vi "OpenProject1.vi"() -> ()   [LabVIEW 2020]
uses:
  <vilib>/Wiresmith Technology/G CLI/CLI Class/CLI.lvclass
  <vilib>/addons/_JKI Toolkits/Caraya/classes/Test Runner/Test Runner.lvclass/Test Runner.ctl
  <vilib>/Wiresmith Technology/G CLI/CLI Class/Output.ctl
  <vilib>/addons/_JKI Toolkits/Caraya/classes/Test Report.JUnit/Test Report.JUnit.lvclass
  C:/Program Files/National Instruments/LabVIEW 2020/vi.lib/addons/_JKI Toolkits/Caraya/classes/Test Report/Test Report.lvclass
  <vilib>/addons/_JKI Toolkits/Caraya/classes/Test Runner.Project/Test Runner.Project.lvclass
  C:/Program Files/National Instruments/LabVIEW 2020/vi.lib/addons/_JKI Toolkits/Caraya/classes/Test Runner/Test Runner.lvclass
  <vilib>/addons/_JKI Toolkits/Caraya/classes/Test Suite/Define Test Suite (Default).vi
  <vilib>/addons/_JKI Toolkits/Caraya/classes/Test Suite/Test Suite.lvclass
  <vilib>/addons/_JKI Toolkits/Caraya/classes/Test Runner/Test Runner.lvclass
  C:/Program Files/National Instruments/LabVIEW 2020/vi.lib/addons/_JKI Toolkits/Caraya/classes/Test Report.JUnit/Test Report.JUnit.lvclass
panel:
  in  "Report Path":path
  in  "Error in":errorcluster
  in  "CLI":refnum<class "CLI.lvclass">
  in  "Project Reference":refnum<vi>
  in  "Virtual Folder (empty: \"My Computer\")":string
  out "Error out":errorcluster
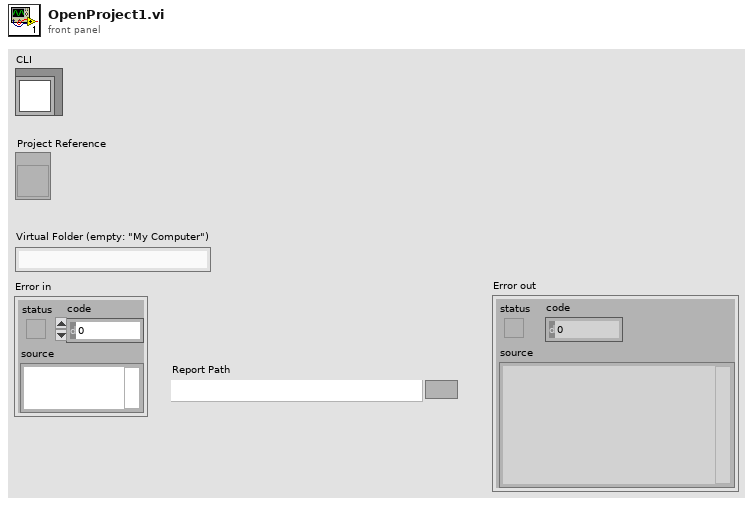
[diagram p1: front panel]
types:
  T1 = typedef "CLI.lvclass/Output.ctl" = enum16{"StdOut", "StdErr"}
  T2 = typedef "Caraya.lvlib/Test Suite.lvclass/Suite PublicEvents -- cluster.ctl" = cluster{"Test Suite Result Event":refnum<user-event>, "suite destroyed":refnum<user-event>, "Test Registration Event":refnum<user-event>, "Assertion Event":refnum<user-event>, "Assertion Update Event":refnum<user-event>}
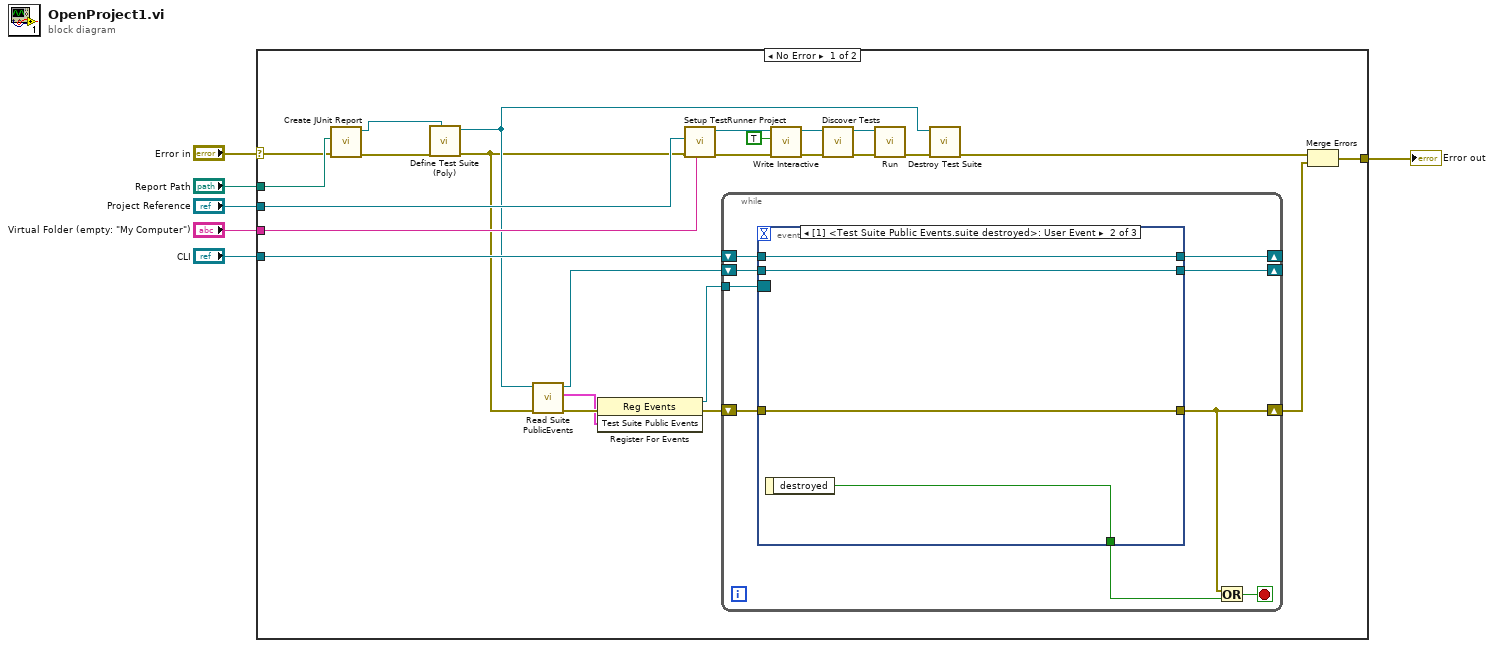
[diagram p0: block diagram]
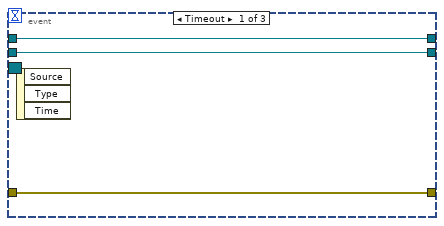
[diagram p2: hidden frame]
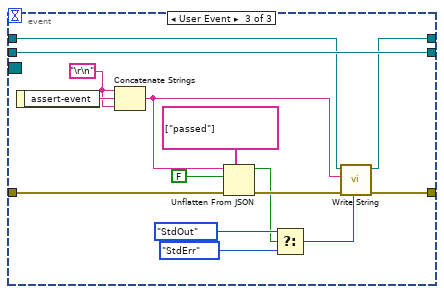
[diagram p3: hidden frame]
diagram:
  n1 = case shown="No Error" "Error in" {
    selector: "Error in" -> [w10 w62]
    tunnel: "Virtual Folder (empty: \"My Computer\")" -> [w26 _]
    tunnel: "Project Reference" -> [w23 _]
    tunnel: "CLI" -> [w18 _]
    tunnel: [w13 w62] -> w3
    tunnel: "Report Path" -> [w11 _]
    frame No Error {
      n2 = call <vilib>:"Create JUnit Report.vi"("error in (no error)"=w10, "Report Path"=w11) -> ("error out"=w9:errorcluster, "Test Report.JUnit out"=w8:refnum<class "Test Report.JUnit.lvclass">)  [unwired: 8 in]
      n3 = call-poly <vilib>:"Define Test Suite (Poly).vi"("Test Report (optional)"=w8, "error in (no error)"=w9) -> ("error out"=w7:errorcluster, "Test Suite"=w14:refnum<class "Test Suite.lvclass">)  [unwired: 8 in]
      n4 = call <vilib>:"Read Suite PublicEvents.vi"("error in (no error)"=w7, "Test Suite in"=w14) -> ("error out"=w22:errorcluster, "Test Suite Public Events"=w20:T2, "Test Suite out"=w15:refnum<class "Test Suite.lvclass">)  [unwired: 7 in]
      n5 = register-events(error in=w22, w20) -> (reference out=w19:refnum<event-registration>, error out=w21:errorcluster)  [unwired: 1 in]
      n6 = call <vilib>:"Setup TestRunner Project.vi"("Virtual Folder (empty: \"My Computer\")"=w26, "error in (no error)"=w7, "Project Refnum"=w23) -> ("error out"=w30:errorcluster, "Test Runner.Project out"=w28:refnum<class "Test Runner.Project.lvclass">)  [unwired: 7 in]
      n7 = while {
        shift-right: [w33] -> w12
        shift-left: w21 -> [w39]
        tunnel: w19 -> [w36]
        shift-right: [w31] -> _
        shift-left: w18 -> [w32]
        shift-right: [w38] -> _
        shift-left: w15 -> [w37]
        stop <- w35 stop-if-true
        n8 = event shown="[1] <Test Suite Public Events.suite destroyed>: User Event" {
          selector: w36 -> [_ _ _]
          dyn-events: _ -> [_ _ _]
          timeout: _ -> [_ _ _]
          tunnel: [w42 w44 w60] -> w33
          tunnel: w39 -> [w42 w44 w53]
          tunnel: [w41 w45 w61] -> w38
          tunnel: w37 -> [w41 w45 w61]
          tunnel: [_ w46 _] -> w34
          tunnel: w32 -> [w40 w43 w59]
          tunnel: [w40 w43 w58] -> w31
          event Timeout {
            n9 = event-data() -> ()  [unwired: 1 in, 3 out]
          }
          event User Event {
            n10 = event-data() -> ("destroyed"=w46:bool)  [unwired: 1 in]
          }
          event User Event {
            w56 = "\r\n"
            n11 = event-data() -> ("assert-event"=w57:string)  [unwired: 1 in]
            n12 = Concatenate Strings(w56, w57, w56) -> (w51:string)
            n13 = Unflatten From JSON(path=string[] ["passed"], JSON string=w51, type and defaults=FALSE, error in (no error)=w53) -> (value=w48:bool, error out=w52:errorcluster)  [unwired: 3 in]
            n14 = Select(t=Output."StdOut" ("Output (StdOut)"), s=w48, f=Output."StdErr" ("Output (StdOut)")) -> (s? t:f=w49:T1)
            n15 = call <vilib>:"Write String.vi"("Output (StdOut)"=w49, "error in (no error)"=w52, "Text to Write"=w51, "CLI in"=w59) -> ("error out"=w60:errorcluster, "CLI out"=w58:refnum<class "CLI.lvclass">)  [unwired: 6 in]
          }
        }
        n16 = Or(x=w33, y=w34) -> (x .or. y?=w35:bool)
      }
      n17 = call <vilib>:"Write Interactive.vi"("Interactive"=TRUE, "Test Runner in"=w28) -> ("Test Runner out"=w27:refnum<class "Test Runner.Project.lvclass">)  [unwired: 9 in]
      n18 = call <vilib>:"Discover Tests.vi"("error in (no error)"=w30, "Test Runner in"=w27) -> ("error out"=w24:errorcluster, "Test Runner out"=w25:refnum<class "Test Runner.Project.lvclass">)  [unwired: 8 in]
      n19 = call <vilib>:"Run.vi"("error in (no error)"=w24, "Test Runner in"=w25) -> ("error out"=w17:errorcluster)  [unwired: 7 in, 2 out]
      n20 = call-dynamic "Destroy Test Suite.vi"("error in (no error)"=w17, "Test Suite in"=w14) -> ("error out"=w16:errorcluster)  [unwired: 8 in, 1 out]
      n21 = Merge Errors(w16, w12) -> (w13:errorcluster)
    }
    frame Error {
    }
  }
  "Error out" <- w3
